vi "Begin.vi"(8 "error in":errorcluster) -> (0 "error out":errorcluster)   [LabVIEW 2017]
doc: "Called before other user functions, this VI can be used to open I/O refnums, load in file data, and do general program initialization. Notice that the <B>error out</B> terminal is simply used for data flow. Wiring it to other structures or subVIs ensures that this VI runs first."
uses:
  <vilib>/Rock Robotics/WPI/DriverStation/WPI_DriverStationRobotMode2.ctl
  <vilib>/Rock Robotics/WPI/Joystick/WPI_JoystickDeviceEnum.ctl
  Robot Global Data.vi
  <vilib>/Rock Robotics/Network Tables/NT Write String Array.vi
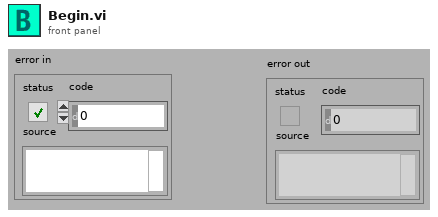
[diagram p1: front panel]
types:
  T1 = typedef "WPI_JoystickDeviceEnum.ctl" = enum16{"USB 0", "USB 1", "USB 2", "USB 3", "USB 4", "USB 5"}
  T2 = typedef "WPI_DriverStationRobotMode2.ctl" = enum16{"Autonomous Disabled", "Autonomous Enabled", "Teleop Disabled", "Teleop Enabled", "Disconnected", "Finish", "Test Disabled", "Test Enabled", "Emergency Stopped"}
  T3 = typedef "WPI_JoystickDevRef.ctl" = cluster{"Device":T1}
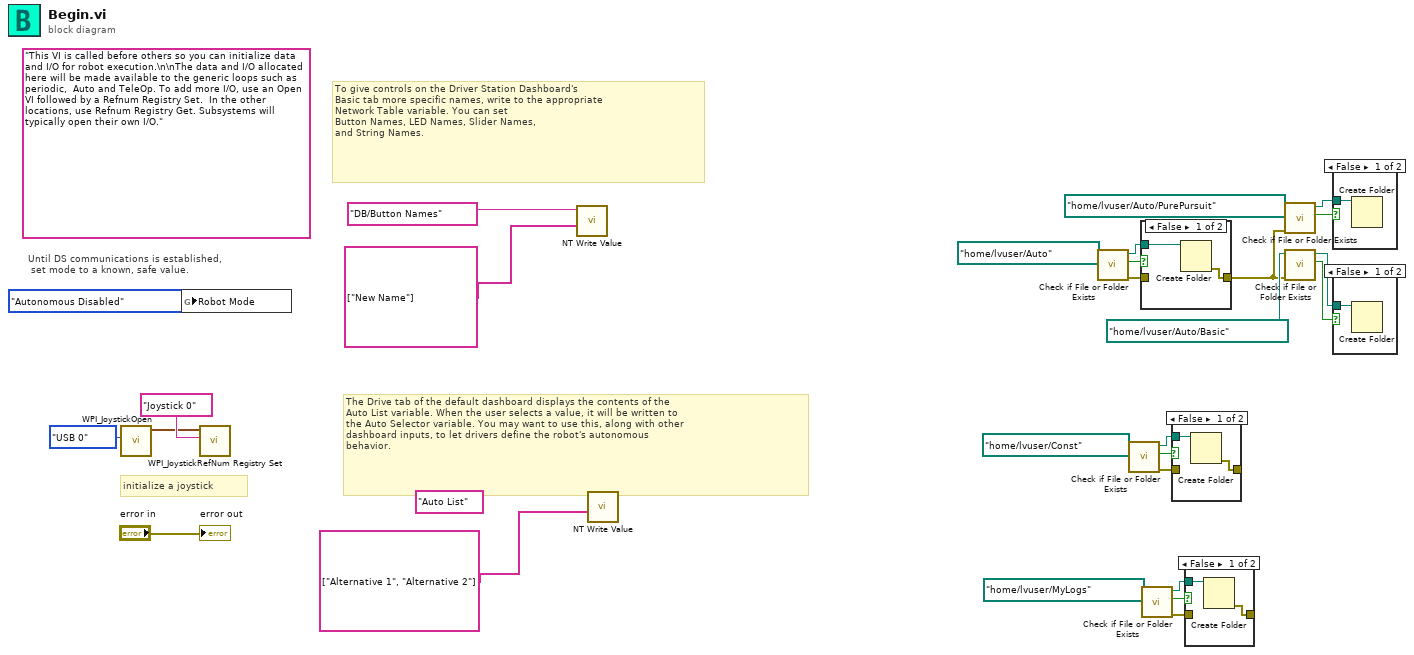
[diagram p0: block diagram]
diagram:
  (unwired) "This VI is called before others so you can initialize data and I/O for robot execution.\n\nThe data and I/O allocated here will be made available to the generic loops such as periodic,  Auto and TeleOp. To add more I/O, use an Open VI followed by a Refnum Registry Set.  In the other locations, use Refnum Registry Get. Subsystems will typically open their own I/O."
  # "The Drive tab of the default dashboard displays the contents of the\nAuto List variable. When the user selects a value, it will be written to\nthe Auto Selector variable. You may want to use this, along with other\ndashboard inputs, to let drivers define the robot's autonomous\nbehavior."
  # "To give controls on the Driver Station Dashboard's\nBasic tab more specific names, write to the appropriate\nNetwork Table variable. You can set\nButton Names, LED Names, Slider Names,\nand String Names."
  # "initialize a joystick"
  # "Until DS communications is established,\n set mode to a known, safe value."
  n1 = call <vilib>:"WPI_JoystickOpen.vi"("JoystickDevice"=WPI_JoystickDeviceEnum."USB 0") -> ("JoystickDevRef"=w26:T3)  [unwired: 10 in]
  n2 = global write "Robot Global Data.vi" "Robot Mode"(WPI_DriverStationRobotMode2."Autonomous Disabled" ("Robot Mode")) -> ()
  n3 = call <vilib>:"WPI_JoystickRefNum Registry Set.vi"("refnum name"="Joystick 0", "JoystickDevRef"=w26) -> ()  [unwired: 8 in, 2 out]
  n4 = call-poly <vilib>:"NT Write Value.vi"("String Array"=string[] ["New Name"], "Name"="DB/Button Names") -> ()  [unwired: 9 in, 1 out]
  n5 = call-poly <vilib>:"NT Write Value.vi"("String Array"=string[] ["Alternative 1", "Alternative 2"], "Name"="Auto List") -> ()  [unwired: 9 in, 1 out]
  n6 = call <vilib>:"Check if File or Folder Exists.vi"("path"=path "/home/lvuser/Auto") -> ("error out"=w19:errorcluster, "file or folder exists?"=w18:bool, "dup path"=w17:path)  [unwired: 8 in]
  n7 = call <vilib>:"Check if File or Folder Exists.vi"("path"=path "/home/lvuser/Const") -> ("error out"=w5:errorcluster, "file or folder exists?"=w6:bool, "dup path"=w7:path)  [unwired: 8 in]
  n8 = case shown="False" w18 {
    tunnel: w17 -> [w30 _]
    tunnel: [w29 w31] -> w9
    tunnel: w19 -> [_ w31]
    frame False {
      n9 = Create Folder(path (use dialog)=w30) -> (error out=w29:errorcluster)  [unwired: 2 in, 2 out]
    }
    frame True {
    }
  }
  n10 = call <vilib>:"Check if File or Folder Exists.vi"("path"=path "/home/lvuser/MyLogs") -> ("error out"=w4:errorcluster, "file or folder exists?"=w3:bool, "dup path"=w2:path)  [unwired: 8 in]
  n11 = case shown="False" w6 {
    tunnel: w7 -> [w33 _]
    tunnel: [w32 w34] -> _
    tunnel: w5 -> [_ w34]
    frame False {
      n12 = Create Folder(path (use dialog)=w33) -> (error out=w32:errorcluster)  [unwired: 2 in, 2 out]
    }
    frame True {
    }
  }
  n13 = case shown="False" w3 {
    tunnel: w2 -> [w36 _]
    tunnel: [w35 w37] -> _
    tunnel: w4 -> [_ w37]
    frame False {
      n14 = Create Folder(path (use dialog)=w36) -> (error out=w35:errorcluster)  [unwired: 2 in, 2 out]
    }
    frame True {
    }
  }
  n15 = call <vilib>:"Check if File or Folder Exists.vi"("error in (no error)"=w9, "path"=path "/home/lvuser/Auto/PurePursuit") -> ("file or folder exists?"=w15:bool, "dup path"=w14:path)  [unwired: 7 in, 1 out]
  n16 = call <vilib>:"Check if File or Folder Exists.vi"("error in (no error)"=w9, "path"=path "/home/lvuser/Auto/Basic") -> ("file or folder exists?"=w11:bool, "dup path"=w12:path)  [unwired: 7 in, 1 out]
  n17 = case shown="False" w15 {
    tunnel: w14 -> [w38 _]
    frame False {
      n18 = Create Folder(path (use dialog)=w38) -> ()  [unwired: 2 in, 3 out]
    }
    frame True {
    }
  }
  n19 = case shown="False" w11 {
    tunnel: w12 -> [w39 _]
    frame False {
      n20 = Create Folder(path (use dialog)=w39) -> ()  [unwired: 2 in, 3 out]
    }
    frame True {
    }
  }
  "error out" <- "error in"
